vi "DVR w Classes Demo.vi"() -> ()   [LabVIEW 2010, in "MyClass.lvclass"]
uses:
  MyClass.lvclass
  MyClass.lvclass/MyClass.ctl
panel:
  out "error out":errorcluster
  out "Numeric":dbl
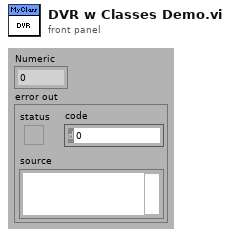
[diagram p1: front panel]
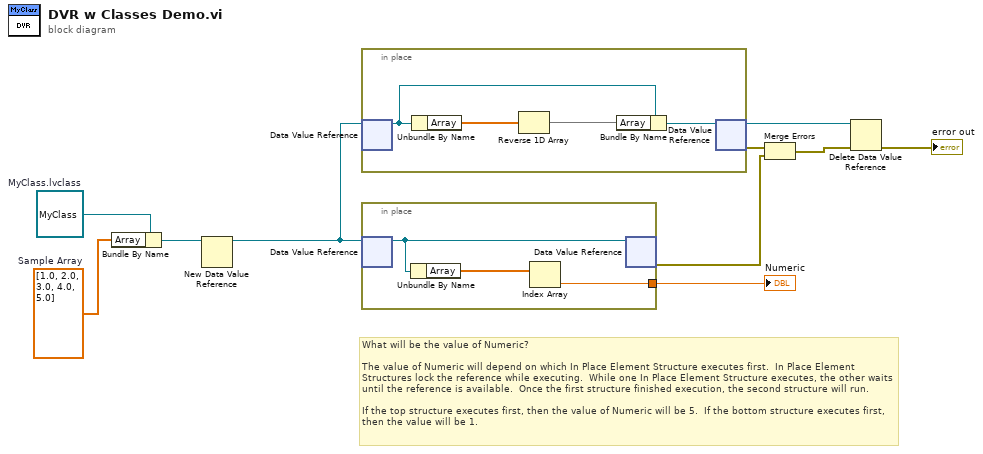
[diagram p0: block diagram]
diagram:
  w7 = dbl[] [1.0, 2.0, 3.0, 4.0, 5.0]  # Sample Array
  w9 = refnum<class "MyClass.lvclass"> refnum  # MyClass.lvclass
  # "What will be the value of Numeric?\n\nThe value of Numeric will depend on which In Place Element Structure executes first.  In Place Element Structures lock the reference while executing.  While one In Place Element Structure executes, the other waits until the reference is available.  Once the first structure finished execution, the second structure will run.\n\nIf the top structure executes first, then the value of Numeric will be 5.  If the bottom structure executes first, then the value will be 1."
  n1 = Bundle By Name "Bundle By Name"(cluster=w9, "Array"=w7) -> (w8:refnum<class "MyClass.lvclass">)
  n2 = New Data Value Reference(data value=w8) -> (data value reference=w10:refnum<data-value>)  [unwired: 1 in, 1 out]
  n3 = in-place "In Place Element Structure" {
    n4 = in-place-dvr #1(w10) -> (w13:refnum<class "MyClass.lvclass">)  [unwired: 1 out]
    n5 = Unbundle By Name "Unbundle By Name"(w13) -> ("Array"=w14:dbl[])
    n6 = Reverse 1D Array(array=w14) -> (reversed array=w12:dbl[])
    n7 = Bundle By Name "Bundle By Name"(cluster=w13, "Array"=w12) -> (w11:refnum<class "MyClass.lvclass">)
    n8 = in-place-dvr #1(w11) -> (w2:refnum<data-value>, w4:errorcluster)
  }
  n9 = in-place "In Place Element Structure" {
    in-place-border: [w15] -> w6
    n10 = in-place-dvr #2(w10) -> (w16:refnum<class "MyClass.lvclass">)  [unwired: 1 out]
    n11 = Unbundle By Name "Unbundle By Name"(w16) -> ("Array"=w17:dbl[])
    n12 = Index Array "Index Array"(array=w17) -> (element=w15:dbl)  [unwired: 1 in]
    n13 = in-place-dvr #2(w16) -> (w5:errorcluster)  [unwired: 1 out]
  }
  "Numeric" <- w6
  n14 = Merge Errors "Merge Errors"(w4, w5) -> (w3:errorcluster)
  n15 = Delete Data Value Reference(data value reference=w2, error in=w3) -> (error out=→"error out":errorcluster)  [unwired: 1 out]
